vi "Create New VI or CTL From Template.vi"(8 "error in":errorcluster, 9 "Block Diagram Preview (Subpanel Ref)":refnum<vi>, 10 "Selected Template VI or CTL name (including file extension)":string, 11 "Destination Folder":path) -> (0 "error out":errorcluster, 3 "Reference of newly created VI":refnum<vi>)   [LabVIEW 2021]
doc: "Creates a new VI or CTL as a \"Save as...\" copy of a template."
panel:
  # "Development\ncontrols/indicators useful for development and testing, but which are not outputs of the VI"
  # "Input\nInputs to the VI"
  # "Output\nOutputs of the VI"
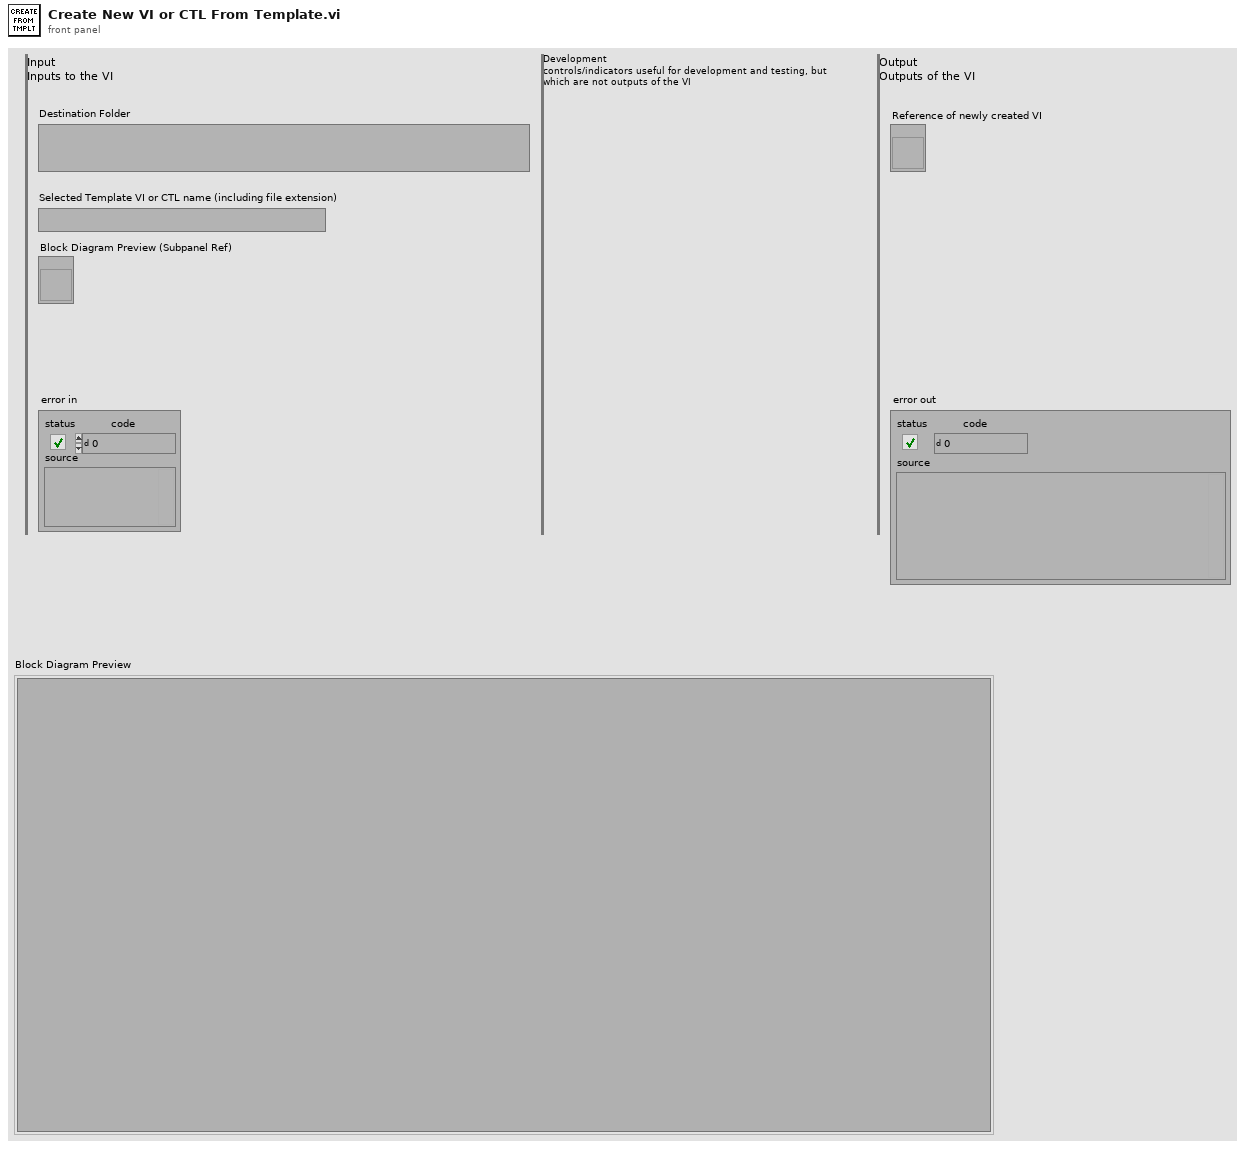
[diagram p1: front panel]
types:
  T1 = enum32{"invalid VI type", "Standard VI", "Control VI", "Global VI", "Polymorphic VI", "Configuration VI", "SubSystem", "Facade VI", "Method VI", "Statechart Diagram VI"}
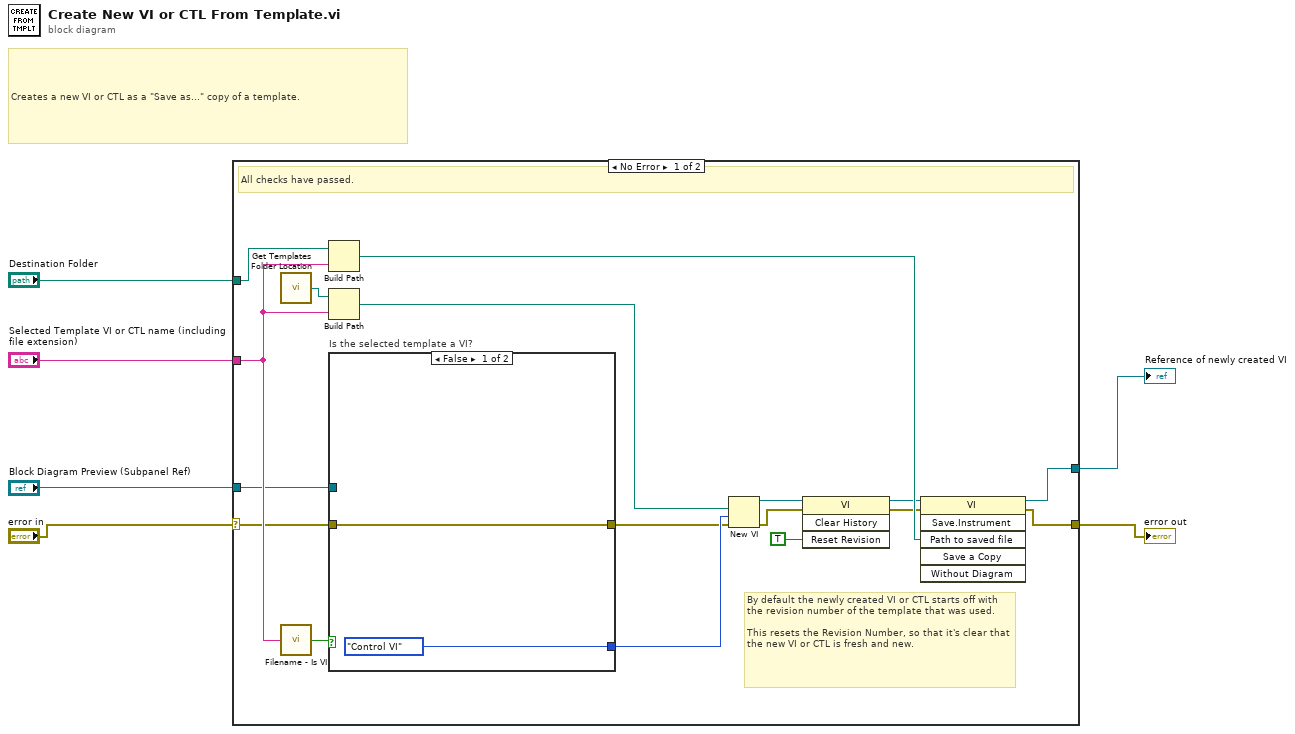
[diagram p0: block diagram]
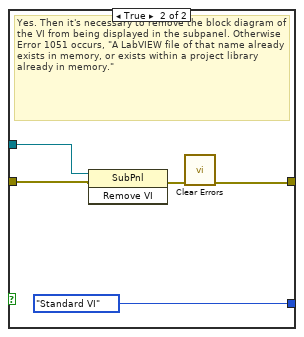
[diagram p2: hidden frame]
diagram:
  # "Creates a new VI or CTL as a \"Save as...\" copy of a template."
  n1 = case shown="No Error" "error in" {
    selector: "error in" -> [w9 w31]
    tunnel: [w20 w31] -> w5
    tunnel: "Selected Template VI or CTL name (including file extension)" -> [w17 _]
    tunnel: "Destination Folder" -> [w23 _]
    tunnel: [w10 _] -> w2
    tunnel: "Block Diagram Preview (Subpanel Ref)" -> [w7 _]
    frame No Error {
      # "By default the newly created VI or CTL starts off with the revision number of the template that was used.\n\nThis resets the Revision Number, so that it's clear that the new VI or CTL is fresh and new."
      # "All checks have passed."
      n2 = call "Get Templates Folder Location.vi"() -> ("Templates Folder Location"=w22:path)
      n3 = call "Filename - Is VI.vi"("Filename (including file extension)"=w17) -> ("Is VI?"=w16:bool)
      n4 = Build Path(base path=w23, name or relative path=w17) -> (appended path=w19:path)
      n5 = Build Path(base path=w22, name or relative path=w17) -> (appended path=w21:path)
      n6 = case "Is the selected template a VI?" shown="False" w16 {
        tunnel: [T1."Control VI" ("vi type (standard vi)") T1."Standard VI" ("vi type (standard vi)")] -> w18
        tunnel: w9 -> [w24 w29]
        tunnel: [w24 w26] -> w8
        tunnel: w7 -> [_ w27]
        frame False {
        }
        frame True {
          # "Yes. Then it's necessary to remove the block diagram of the VI from being displayed in the subpanel. Otherwise Error 1051 occurs, \"A LabVIEW file of that name already exists in memory, or exists within a project library already in memory.\""
          n7 = invoke on="Invoke Node" class="SubPnl" method="Remove VI"(reference=w27, error in=w29) -> (error out=w28:errorcluster)  [unwired: 1 in, 2 out]
          n8 = call <vilib>:"Clear Errors.vi"("error in (no error)"=w28) -> ("error out"=w26:errorcluster)  [unwired: 5 in, 1 out]
        }
      }
      n9 = New VI(8:w8, 9:w18, 10:w21) -> (0:w14:errorcluster, 3:w15:refnum<vi>)  [unwired: 4 in]
      n10 = invoke class="VI" method="Clear History"(reference=w15, error in=w14, "Reset Revision"=TRUE) -> (reference out=w12:refnum<vi>, error out=w13:errorcluster)  [unwired: 1 in, 2 out]
      n11 = invoke class="VI" method="Save.Instrument"(reference=w12, error in=w13, "Path to saved file"=w19) -> (reference out=w10:refnum<vi>, error out=w20:errorcluster)  [unwired: 3 in, 4 out]
    }
    frame Error {
      # "Do nothing. The error message will be handled later, downstream"
      # "One or more checks failed."
    }
  }
  "error out" <- w5
  "Reference of newly created VI" <- w2
